vi "global_m.vi"() -> ()   [LabVIEW 2018]
panel:
  in  "baud rate":u16=9600
  in  "Speed":dbl=50.0 format="%.3f"
  in  "Backlash compensation":dbl=10.0 format="%.2f"
  in  "Backlash":bool
  in  "Grating, gr/mm":u16(ring)=2 items=["2400", "1800", "1200", "600", "300", "150"]
  in  "Delay Before\nread (ms)":u32=50
  in  "Calibration, nm":dbl=265.0 format="%2.2f"
  in  "VISA resource name":refnum<visa-resource-name>="COM2"
  # "Backlash \nCompensation, nm"
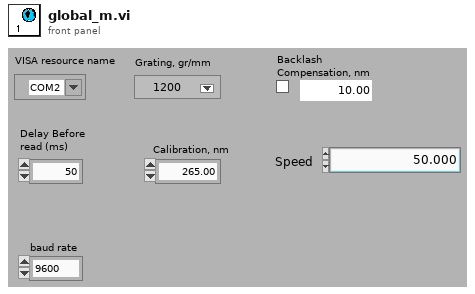
[diagram p1: front panel]
diagram:
